vi "get senserdata.vi"(10 "senser name":string, 11 "configtable":T7 {"CHS"."display" format="%b"}) -> (0 "CAl":T6, 1 "sensers data":string[](array[string]), 2 "chanel":T1={"chanel"="", "ch name"="", "Enable"=FALSE, "sensors"="", "signal type"="", "unit"="", "K"=0.0, "B"=0.0, "ALarm"=FALSE, "CAl"={"manner"=enum."线性", "data"=[]}, "Fre"=0.0, "type"=enum."volet", "Gain"=enum."±10V", "Filter"={"en"=FALSE, "value"=0, "Boolean"=FALSE}, "Power"={"power_en"=FALSE, "Mode"=enum."电压", "value"=0.0, "Boolean"=FALSE}})   [LabVIEW 2011]
uses:
  signal type.ctl
  gain.ctl
  single chanel.ctl
  filter.ctl
  Power_config.ctl
  singlechtype.ctl
  CHS.ctl
  contable.ctl
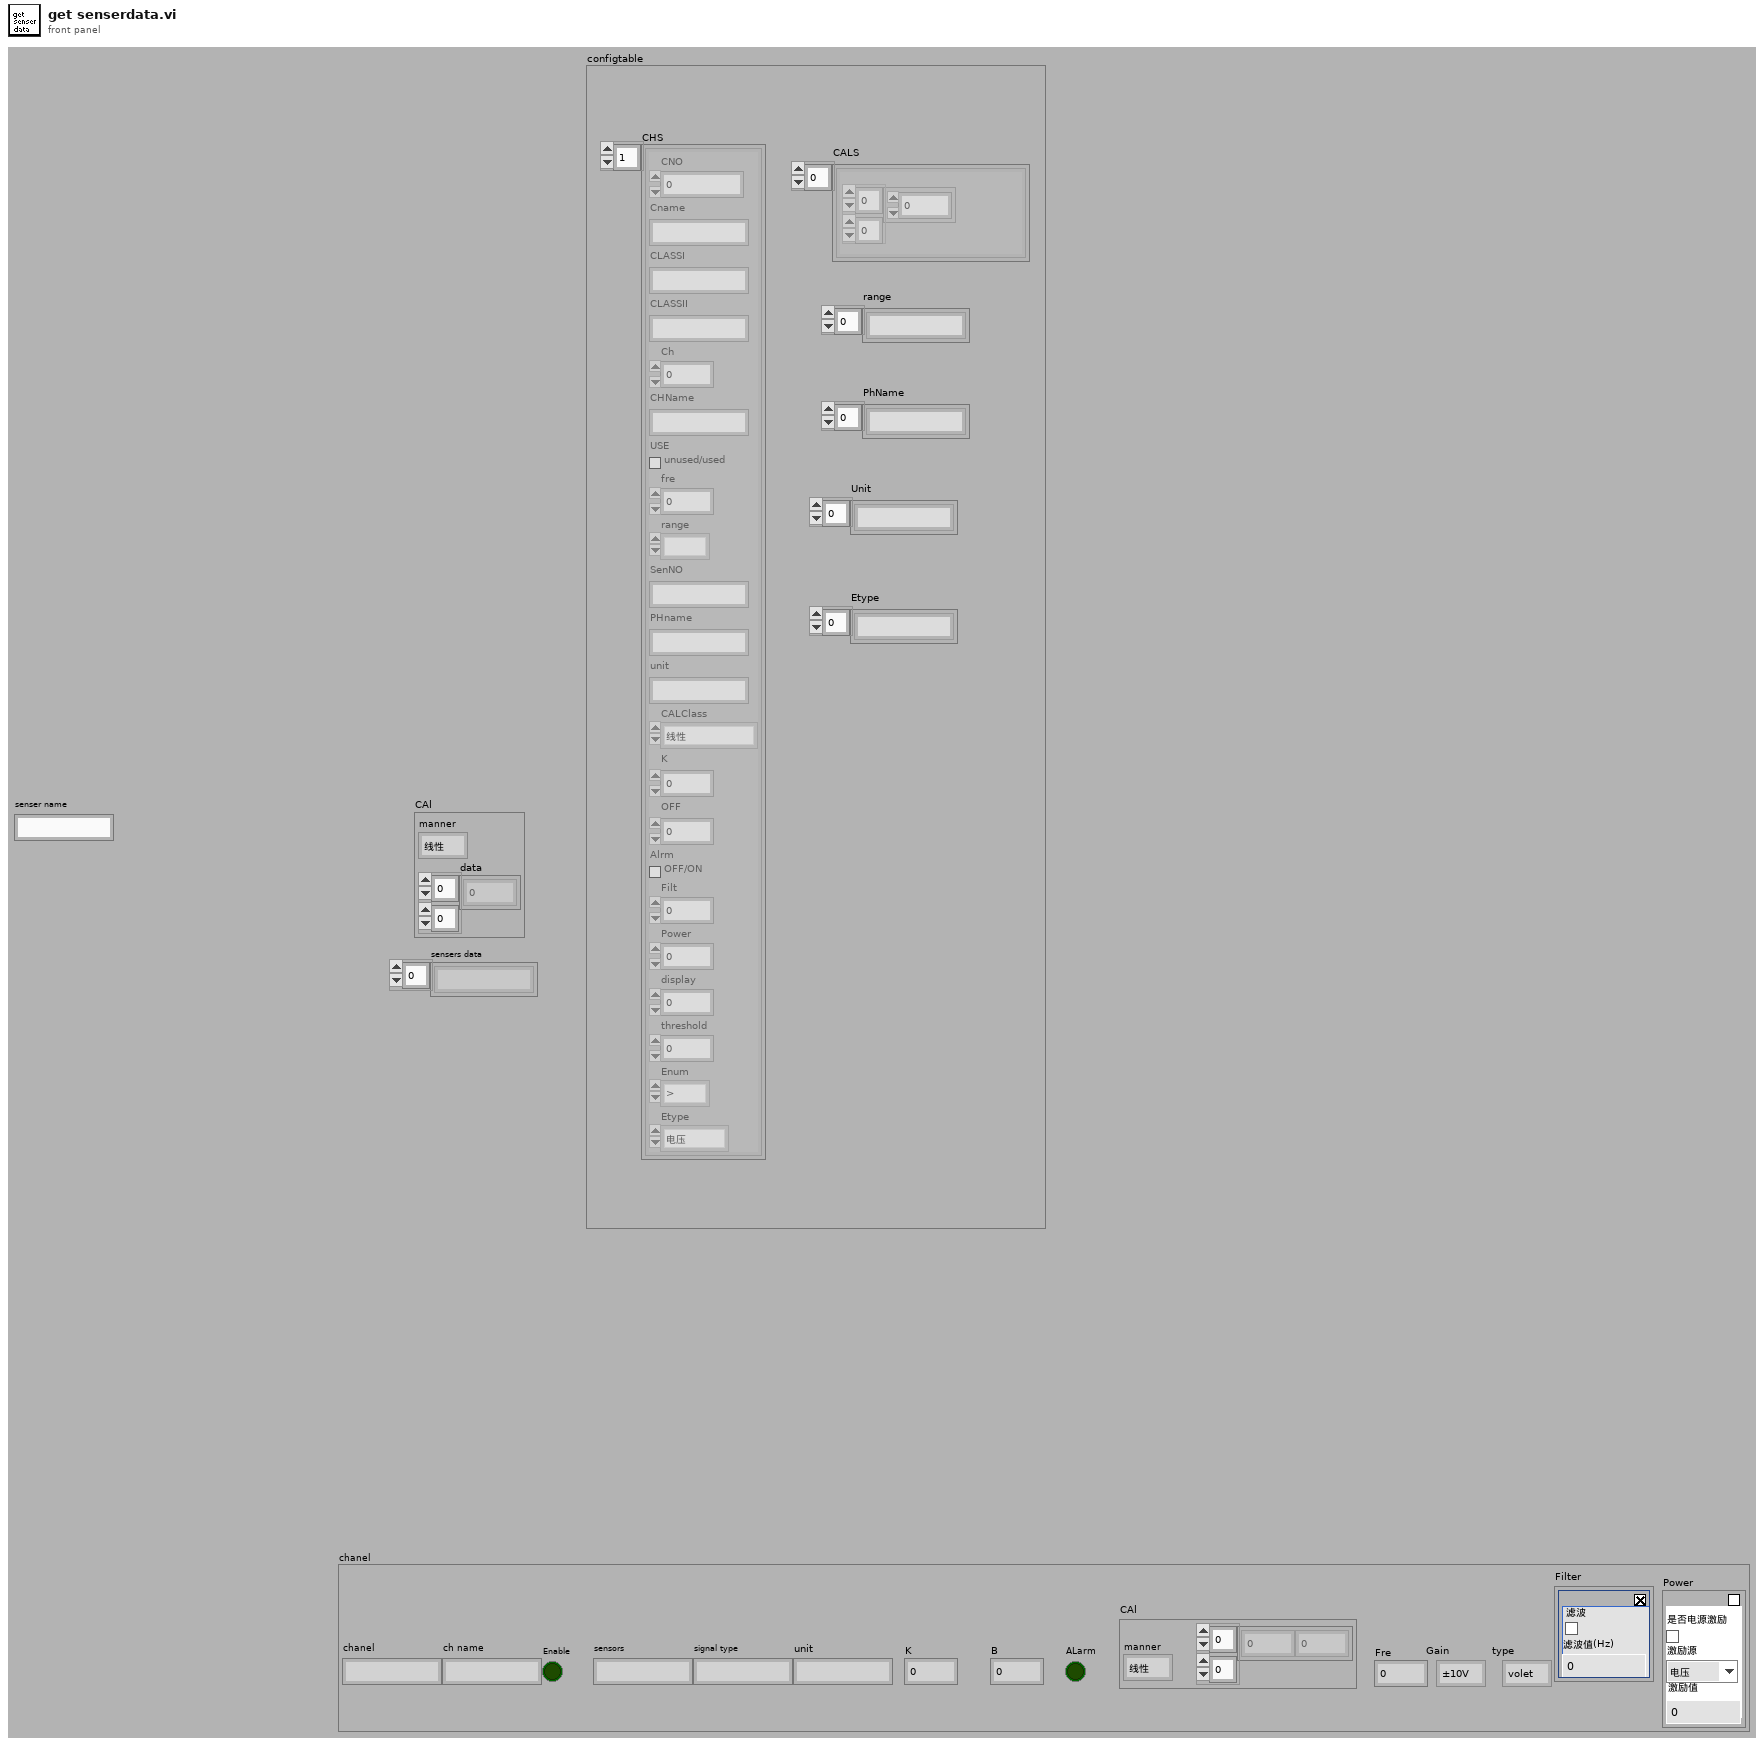
[diagram p1: front panel]
types:
  T1 = typedef "single chanel.ctl" = cluster{"chanel":string, "ch name":string, "Enable":bool, "sensors":string, "signal type":string, "unit":string, "K":dbl, "B":dbl, "ALarm":bool, "CAl":cluster{"manner":enum16{"线性", "查表"}, "data":dbl[][]}, "Fre":dbl, "type":T2, "Gain":T3, "Filter":T4, "Power":T5}
  T2 = typedef "signal type.ctl" = enum16{"未设置", "volet", "current", "vibration", "electric charge ", "resistance "}
  T3 = typedef "gain.ctl" = enum16{"±10V", "±5V", "±2.5V", "±1V", "±500mV", "±100mV", "10V", "5V", "2.5V", "1V", "500mV", "100mV"}
  T4 = typedef "filter.ctl" = cluster{"en":bool, "value":i32, "Boolean":bool}
  T5 = typedef "Power_config.ctl" = cluster{"power_en":bool, "Mode":enum16{"电压", "电流"}, "value":dbl, "Boolean":bool}
  T6 = cluster{"manner":enum16{"线性", "查表"}, "data":dbl[][]}
  T7 = typedef "contable.ctl" = cluster{"CHS":T8, "CALS":cluster{"Array":dbl[][]}[], "range":string[], "PhName":string[], "Unit":string[], "Etype":string[]}
  T8 = typedef "CHS.ctl" = T9[]
  T9 = typedef "singlechtype.ctl" = cluster{"CNO":u8, "Cname":string, "CLASSI":string, "CLASSII":string, "Ch":u8, "CHName":string, "USE":bool, "fre":dbl, "range":enum16{""}, "SenNO":string, "PHname":string, "unit":string, "CALClass":enum8{"线性", "查表", "公式"}, "K":dbl, "OFF":dbl, "Alrm":bool, "Filt":dbl, "Power":u8, "display":u8, "threshold ":dbl, "Enum":enum16{">", ">=", "<", "<=", "<>(在范围内）", "><（在范围外）"}, "Etype":enum16{"电压", "电流", "电阻", "热电偶K", "热电偶T"}}
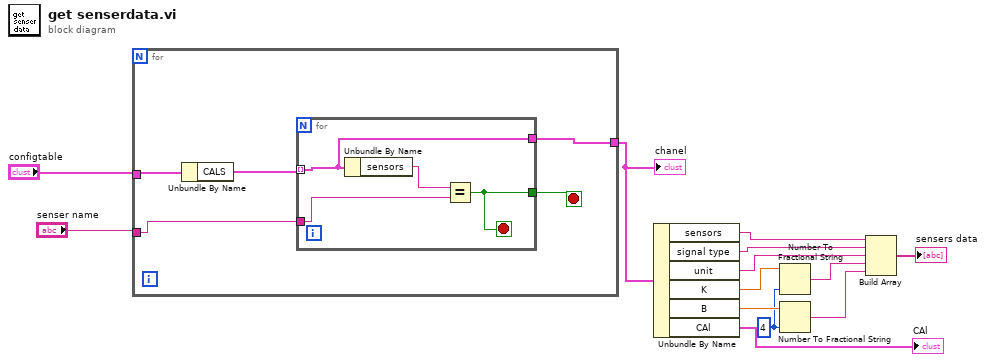
[diagram p0: block diagram]
diagram:
  w2 = i16 4 ("precision (6)")
  n1 = for {
    tunnel: "configtable" -> [w18]
    tunnel: "senser name" -> [w16]
    tunnel: [w15] -> w1
    stop <- w14 stop-if-true
    n2 = Unbundle By Name(w18) -> ("CALS"=w17:cluster{"Array":dbl[][]}[])
    n3 = for {
      tunnel: w17 -> [w20] mode=indexing
      tunnel: w16 -> [w21]
      tunnel: [w20] -> w15
      tunnel: [w19] -> w14
      stop <- w19 stop-if-true
      n4 = Unbundle By Name(w20) -> ("sensors"=w22:string)
      n5 = Equal?(x=w22, y=w21) -> (x = y?=w19:bool)
    }
  }
  "chanel" <- w1
  n6 = Unbundle By Name(w1) -> ("sensors"=w9:string, "signal type"=w8:string, "unit"=w7:string, "K"=w11:dbl, "B"=w10:dbl, "CAl"=→"CAl":T6)
  n7 = Number To Fractional String(number=w11, precision (6)=w2) -> (F-format string=w6:string)  [unwired: 2 out]
  n8 = Number To Fractional String(number=w10, precision (6)=w2) -> (F-format string=w5:string)  [unwired: 2 out]
  n9 = Build Array(w9, w8, w7, w6, w5) -> (→"sensers data":string[])
